vi "CreateFile.vi"(11 "Date/time":string) -> (0 "error out":errorcluster, 3 "Byte Stream File out":refnum<file>)   [LabVIEW 2018]
doc: "Creates the log file. In this VI is where the log file's name is determined."
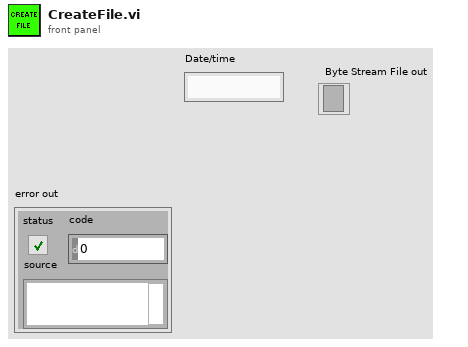
[diagram p1: front panel]
types:
  T1 = typedef "NetComm_MatchType.ctl" = enum32{"None", "Practice", "Qualification", "Elimination"}
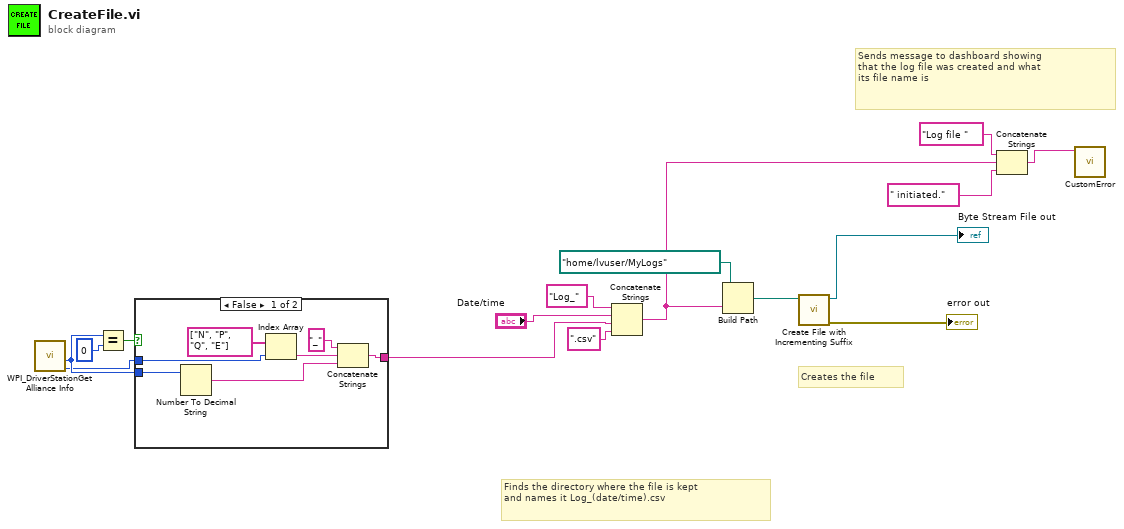
[diagram p0: block diagram]
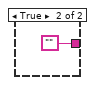
[diagram p2: hidden frame]
diagram:
  # "Finds the directory where the file is kept\nand names it Log_(date/time).csv"
  # "Creates the file"
  # "Sends message to dashboard showing\nthat the log file was created and what \nits file name is"
  n1 = call <vilib>:"WPI_DriverStationGet Alliance Info.vi"() -> ("Match Type"=w1:T1, "Match Number"=w8:u16)  [unwired: 6 in, 4 out]
  n2 = Equal?(x=w8, y=u16 0) -> (x = y?=w10:bool)
  n3 = case shown="False" w10 {
    tunnel: [w22 ""] -> w2
    tunnel: w8 -> [w23 _]
    tunnel: w1 -> [w19 _]
    frame False {
      n4 = Number To Decimal String(number=w23) -> (decimal integer string=w17:string)  [unwired: 1 in]
      n5 = Index Array(array=string[] ["N", "P", "Q", "E"], index=w19) -> (element=w18:string)
      n6 = Concatenate Strings("_" ("string"), w18, w17) -> (w22:string)
    }
    frame True {
    }
  }
  n7 = Concatenate Strings("Log_" ("string"), "Date/time", w2, ".csv" ("string")) -> (w4:string)
  n8 = Build Path(base path=path "/home/lvuser/MyLogs", name or relative path=w4) -> (appended path=w5:path)
  n9 = call <vilib>:"Create File with Incrementing Suffix.vi"("file path"=w5) -> ("error out"=→"error out":errorcluster, "refnum out"=→"Byte Stream File out":refnum<file>)  [unwired: 8 in, 1 out]
  n10 = Concatenate Strings("Log file " ("Source"), w4, " initiated." ("string")) -> (w12:string)
  n11 = call "CustomError.vi"("String"=w12) -> ()  [unwired: 10 in, 1 out]
